vi "Read navX Class.vi"(8 "error in (no error)":errorcluster, 11 "navX in":refnum<class "navX.lvclass">) -> (0 "error out":errorcluster, 2 "navX Library v3.lvlib:navX - Base.lvclass":refnum<class "navX - Base.lvclass">, 3 "navX out":refnum<class "navX.lvclass">)   [LabVIEW 2015, in "navX Library v3.lvlib" / "navX.lvclass"]
uses:
  navX.lvclass
  navX - Base/navX - Base.lvclass
  navX.lvclass/navX.ctl
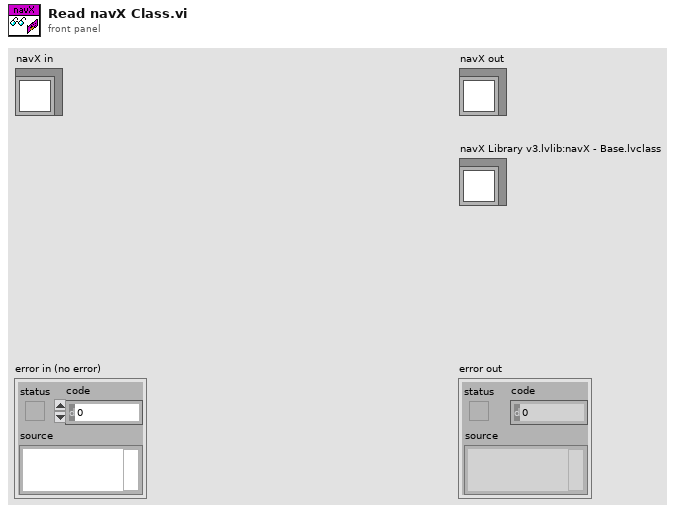
[diagram p1: front panel]
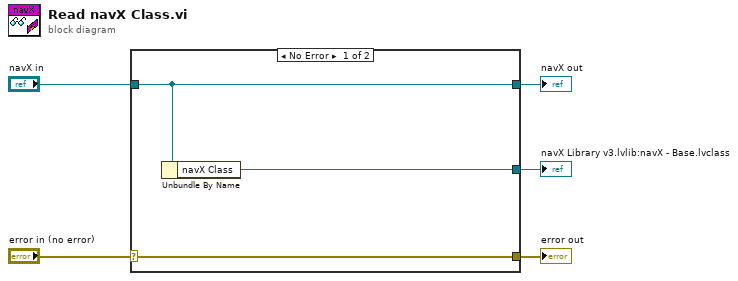
[diagram p0: block diagram]
diagram:
  n1 = case shown="No Error" "error in (no error)" {
    selector: "error in (no error)" -> [w8 w9]
    tunnel: [w8 w9] -> w4
    tunnel: [w7 w10] -> w2
    tunnel: "navX in" -> [w7 w10]
    tunnel: [w6 _] -> w1
    frame No Error {
      n2 = Unbundle By Name(w7) -> ("navX Class"=w6:refnum<class "navX - Base.lvclass">)
    }
    frame Error {
    }
  }
  "error out" <- w4
  "navX out" <- w2
  "navX Library v3.lvlib:navX - Base.lvclass" <- w1
